vi "Add Point.vi"(8 "error in (no error)":errorcluster, 9 "New X":i32, 10 "New Y":i32, 11 "Outline in":refnum<class "Outline.lvclass">) -> (0 "error out":errorcluster, 3 "Outline out":refnum<class "Outline.lvclass">)   [LabVIEW 2013, in "Outline.lvclass"]
uses:
  Outline.lvclass
  Outline.lvclass/Outline.ctl
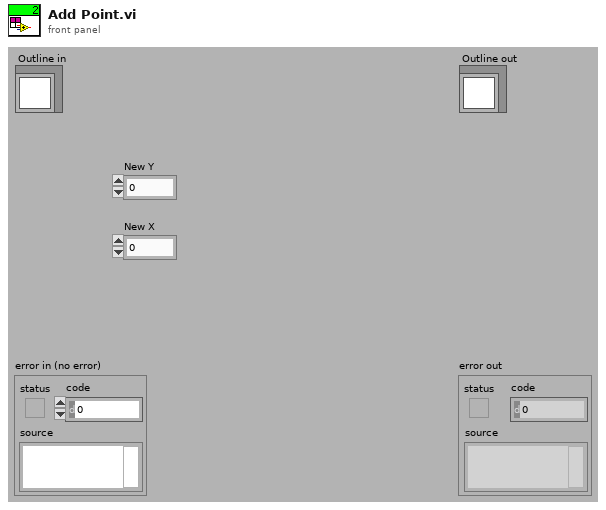
[diagram p1: front panel]
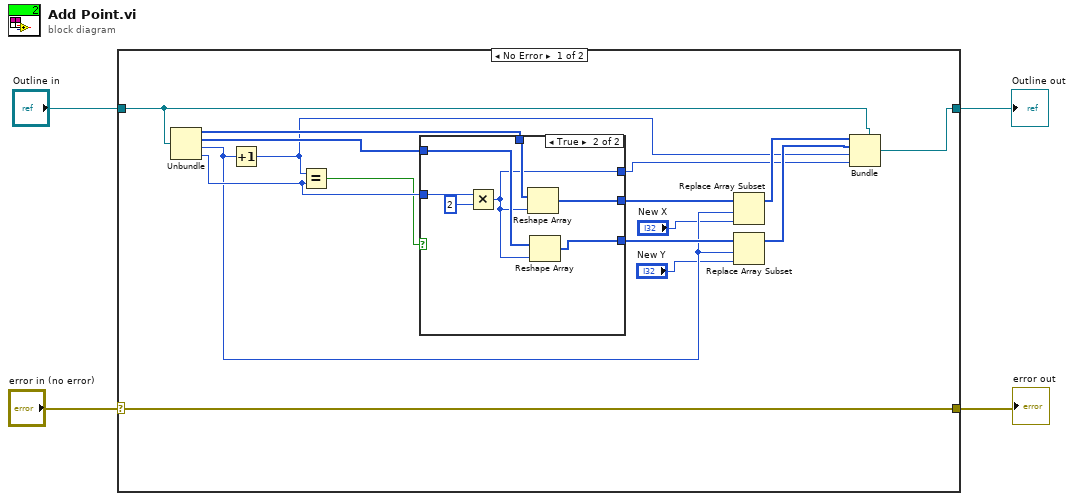
[diagram p0: block diagram]
diagram:
  n1 = case shown="No Error" "error in (no error)" {
    selector: "error in (no error)" -> [w20 w32]
    tunnel: [w20 w32] -> w3
    tunnel: [w14 w31] -> w1
    tunnel: "Outline in" -> [w15 w31]
    frame No Error {
      n2 = Unbundle(w15) -> (w19:i32[], w16:i32[], w11:i32, w18:i32)
      n3 = Increment(x=w11) -> (x+1=w8:i32)
      n4 = Equal?(x=w8, y=w18) -> (x = y?=w17:bool)
      n5 = case shown="True" w17 {
        tunnel: w19 -> [w23 w30]
        tunnel: w18 -> [w21 w29]
        tunnel: w16 -> [w22 w27]
        tunnel: [w23 w26] -> w13
        tunnel: [w22 w25] -> w12
        tunnel: [w21 w24] -> w7
        frame False {
        }
        frame True {
          n6 = Multiply(x=w29, y=2) -> (x*y=w24:i32)
          n7 = Reshape Array(w30, w24) -> (w26:i32[])
          n8 = Reshape Array(w27, w24) -> (w25:i32[])
        }
      }
      n9 = Replace Array Subset(array=w13, new element="New X", index=w11) -> (w10:i32[])
      n10 = Replace Array Subset(array=w12, new element="New Y", index=w11) -> (w9:i32[])
      n11 = Bundle(cluster=w15, w10, w9, w8, w7) -> (w14:refnum<class "Outline.lvclass">)
    }
    frame Error {
    }
  }
  "error out" <- w3
  "Outline out" <- w1
